vi "All Strings.vi"(8 "error in (no error)":errorcluster, 11 "StringGroup in":refnum<class "Group STR.lvclass">) -> (0 "error out":errorcluster, 1 "Timestamps":dbl[](array[numeric]), 2 "Strings":string[](array[string]), 3 "StringGroup out":refnum<class "Group STR.lvclass">)   [LabVIEW 2020, in "Vecto.lvlib" / "Group STR.lvclass"]
uses:
  Group STR.lvclass
  Group STR.lvclass/Group STR.ctl
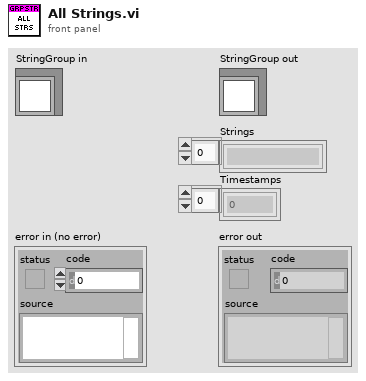
[diagram p1: front panel]
types:
  T1 = typedef "Vecto.lvlib/StringGroup.lvclass/Ref.ctl" = cluster{"Strings":string[], "Timestamp":dbl[]}
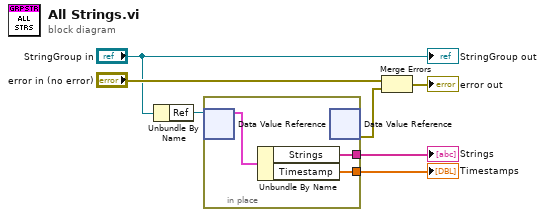
[diagram p0: block diagram]
diagram:
  n1 = Unbundle By Name("StringGroup in") -> ("Ref"=w6:refnum<data-value>)
  n2 = in-place {
    in-place-border: [w9] -> w4
    in-place-border: [w8] -> w1
    n3 = in-place-dvr #1(w6) -> (w10:T1)  [unwired: 1 out]
    n4 = Unbundle By Name(w10) -> ("Strings"=w9:string[], "Timestamp"=w8:dbl[])
    n5 = in-place-dvr #1() -> (w2:errorcluster)  [unwired: 1 in, 1 out]
  }
  "Strings" <- w4
  "Timestamps" <- w1
  n6 = Merge Errors("error in (no error)", w2) -> (→"error out":errorcluster)
  "StringGroup out" <- "StringGroup in"
